vi "Sec-4_Akatsuki.vi"() -> ()   [LabVIEW 2020]
panel:
  in  "Table Control":string[][](table)
  out "Humidity":bool
  out "Temperature":bool
  out "Temperature":dbl(slide) scale=0.0..80.0
  out "Humidity Chart":dbl(graph)
  out "Temperature Chart":dbl(graph)
  out "Humidity":dbl(knob) scale=0.0..100.0
  in  "VISA resource name":refnum<visa-resource-name>
  out "Smoke Chart":dbl(graph)
  out "Smoke":bool
  out "Fire Indicator":bool
  out "Smoke":sgl(slide) scale=0.0..1.0 scale format="%#_1g"
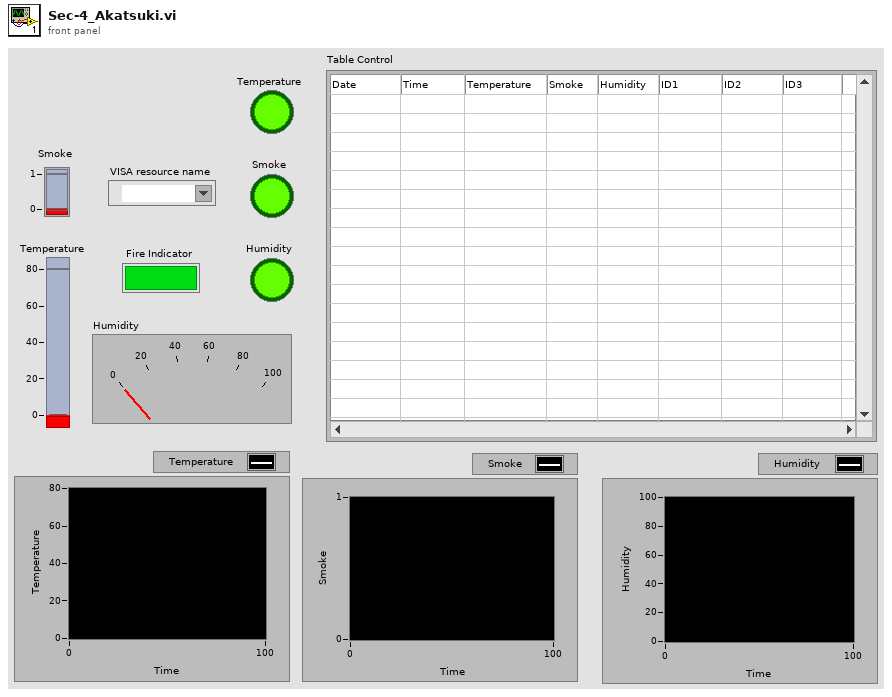
[diagram p1: front panel]
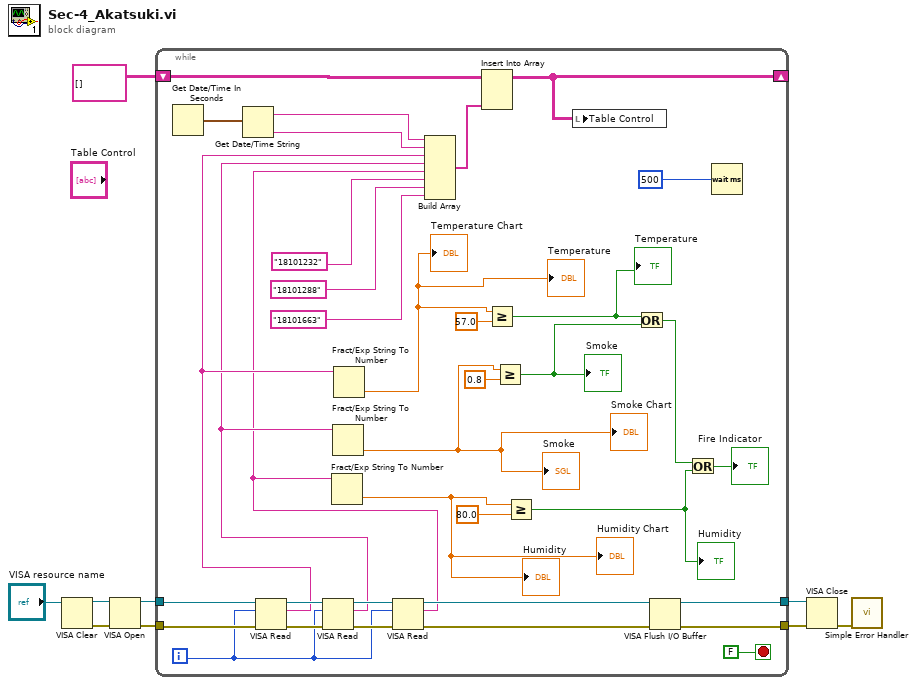
[diagram p0: block diagram]
diagram:
  n1 = VISA Clear(VISA resource name="VISA resource name") -> (VISA resource name out=w9:refnum<visa-resource-name>, error out=w8:errorcluster)  [unwired: 1 in]
  n2 = VISA Open(error in (no error)=w8, VISA resource name=w9) -> (VISA resource name=w7:refnum<visa-resource-name>, error out=w6:errorcluster)  [unwired: 3 in]
  n3 = while {
    tunnel: w7 -> [w45]
    tunnel: w6 -> [w44]
    tunnel: [w41] -> w5
    tunnel: [w40] -> w4
    shift-right: [w37] -> _
    shift-left: string[][] [] -> [w38]
    i -> [w21]
    stop <- FALSE stop-if-true
    n4 = Get Date/Time In Seconds() -> (seconds since 1Jan1904=w36:timestamp)
    n5 = Get Date/Time String(seconds (now)=w36) -> (date string=w35:string, time string=w34:string)  [unwired: 2 in]
    n6 = VISA Read(VISA resource name=w45, byte count=w21, error in (no error)=w44) -> (VISA resource name out=w43:refnum<visa-resource-name>, read buffer=w20:string, error out=w42:errorcluster)  [unwired: 1 out]
    n7 = VISA Read(VISA resource name=w43, byte count=w21, error in (no error)=w42) -> (VISA resource name out=w25:refnum<visa-resource-name>, read buffer=w19:string, error out=w24:errorcluster)  [unwired: 1 out]
    n8 = Fract/Exp String To Number(string=w19) -> (number=w29:dbl)  [unwired: 3 in, 1 out]
    "Smoke Chart" <- w29
    "Smoke" <- w29
    n9 = Fract/Exp String To Number(string=w20) -> (number=w26:dbl)  [unwired: 3 in, 1 out]
    "Temperature" <- w26
    "Temperature Chart" <- w26
    n10 = VISA Read(VISA resource name=w25, byte count=w21, error in (no error)=w24) -> (VISA resource name out=w22:refnum<visa-resource-name>, read buffer=w18:string, error out=w23:errorcluster)  [unwired: 1 out]
    n11 = Fract/Exp String To Number(string=w18) -> (number=w16:dbl)  [unwired: 3 in, 1 out]
    "Humidity" <- w16
    "Humidity Chart" <- w16
    n12 = Build Array(w35, w34, w20, w19, w18, "18101232" ("element"), "18101288" ("element"), "18101663" ("element")) -> (w33:string[])
    n13 = Insert Into Array(array=w38, new element=w33) -> (w37:string[][])  [unwired: 2 in]
    n14 = Greater Or Equal?(x=w26, y=57.0) -> (x >= y?=w27:bool)
    "Temperature" <- w27
    n15 = Greater Or Equal?(x=w29, y=0.8) -> (x >= y?=w28:bool)
    "Smoke" <- w28
    n16 = Greater Or Equal?(x=w16, y=80.0) -> (x >= y?=w15:bool)
    "Humidity" <- w15
    n17 = local write "Table Control"(w37) -> ()
    n18 = Or(x=w27, y=w28) -> (x .or. y?=w14:bool)
    n19 = VISA Flush I/O Buffer(VISA resource name=w22, error in (no error)=w23) -> (VISA resource name out=w41:refnum<visa-resource-name>, error out=w40:errorcluster)  [unwired: 1 in]
    n20 = Or(x=w14, y=w15) -> (x .or. y?=→"Fire Indicator":bool)
    n21 = Wait (ms)(milliseconds to wait=u32 500) -> ()  [unwired: 1 out]
  }
  n22 = VISA Close(VISA resource name=w5, error in (no error)=w4) -> (error out=w3:errorcluster)
  n23 = call <vilib>:"Simple Error Handler.vi"("error in (no error)"=w3) -> ()  [unwired: 4 in, 5 out]
